vi "WPI_DMAClose.vi"(8 "error in (no error)":errorcluster, 11 "DMARef":T1) -> (0 "error out":errorcluster)   [LabVIEW 2017]
doc: "Closes the reference to the DMA stream from the FPGA module of the roboRIO you specify. Use this VI to close each DMA reference that you open with the Open VI.\n\nThis software is licensed. Open the labview\\readme\\WPI Robotics Library Open Source License.txt file for more information."
uses:
  <vilib>/Rock Robotics/WPI/DMA/WPI_DMARef.ctl
  <vilib>/Rock Robotics/SystemInterfaces/DMA/FPGA_DMAWriteConfigOperation.ctl
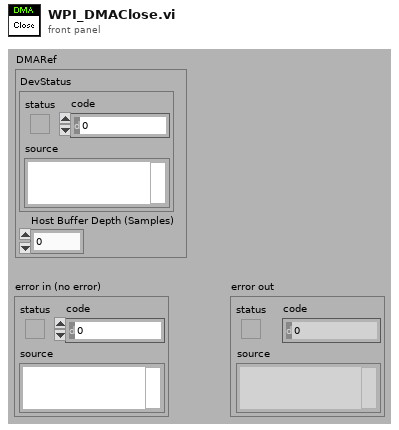
[diagram p1: front panel]
types:
  T1 = typedef "WPI_DMARef.ctl" = cluster{"DevStatus":errorcluster, "Host Buffer Depth (Samples)":u32}
  T2 = typedef "FPGA_DMAWriteConfigOperation.ctl" = enum16{"Update Pause", "Update Enable", "Update SampleClock"}
  T3 = typedef "FPGA_DMADevRef.ctl" = cluster{"DevStatus":errorcluster}
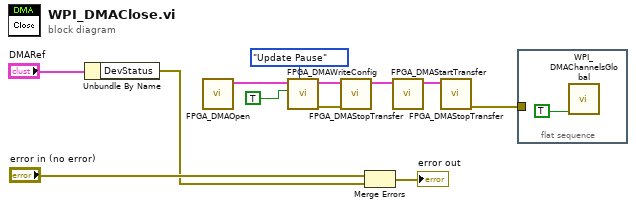
[diagram p0: block diagram]
diagram:
  n1 = Unbundle By Name("DMARef") -> ("DevStatus"=w2:errorcluster)
  n2 = call <vilib>:"FPGA_DMAOpen.vi"() -> ("DMADevRef"=w10:T3)  [unwired: 1 in, 10 out]
  n3 = call <vilib>:"FPGA_DMAWriteConfig.vi"("Operation"=FPGA_DMAWriteConfigOperation."Update Pause", "Pause"=TRUE, "DMADevRef"=w10) -> ("error out"=w7:errorcluster, "DMADevRef"=w8:T3)  [unwired: 3 in, 4 out]
  n4 = call <vilib>:"FPGA_DMAStopTransfer.vi"("error in (no error)"=w7, "DMADevRef In"=w8) -> ("DMADevRef Out"=w5:T3)  [unwired: 9 out]
  n5 = Merge Errors("error in (no error)", w2) -> (→"error out":errorcluster)
  n6 = call <vilib>:"FPGA_DMAStartTransfer.vi"("DMADevRef In"=w5) -> ("DMADevRef Out"=w6:T3)  [unwired: 1 in, 9 out]
  n7 = call <vilib>:"FPGA_DMAStopTransfer.vi"("DMADevRef In"=w6) -> ("error out"=w4:errorcluster)  [unwired: 1 in, 9 out]
  n8 = flat-sequence {
    tunnel: w4 -> [_]
    frame #0 {
      n9 = call <vilib>:"WPI_DMAChannelsGlobal.vi"("Clear"=TRUE) -> ()  [unwired: 3 in, 8 out]
    }
  }
